vi "9203_UI.vi"(8 "error in (no error)":errorcluster, 11 "Node Ptr":T2 format="%.0x") -> (0 "error out":errorcluster)   [LabVIEW 2017, in "Modules.lvlib" / "9203.lvclass"]
uses:
  9203.lvclass
  <vilib>/NI Veristand/Custom Device API/Custom Device Item Ref.ctl
  RSI Module/SubPanel Command.ctl
  C:/Users/dbuck/Documents/GitHub/Scan-Engine-Custom-Device-Classes/Source/RSI Module/RSI Module.lvclass
  9203.lvclass/9203.ctl
  Range.ctl
  RSI Module/RSI Module.lvclass
  <vilib>/NI Veristand/Custom Device API/Custom Device API.lvlib
panel:
  out "_SupportedRanges":string[][](array[string])=[["+/- 20mA", "0-20 mA"], ["+/- 20mA", "0-20 mA"], ["+/- 20mA", "0-20 mA"], ["+/- 20mA", "0-20 mA"], ["+/- 20mA", "0-20 mA"], ["+/- 20mA", "0-20 mA"], ["+/- 20mA", "0-20 mA"], ["+/- 20mA", "0-20 mA"]]
  in  "_Update Chan Settings":bool
  in  "_Update Ring Controls":bool
  in  "_Input Ranges":T1(array[ring])=[enum."+/- 10V", enum."+/- 10V", enum."+/- 10V", enum."+/- 10V", enum."+/- 10V", enum."+/- 10V", enum."+/- 10V", enum."+/- 10V", enum."+/- 10V", enum."+/- 10V", enum."+/- 10V", enum."+/- 10V", enum."+/- 10V", enum."+/- 10V", enum."+/- 10V", enum."+/- 10V", enum."+/- 10V", enum."+/- 10V", enum."+/- 10V", enum."+/- 10V", enum."+/- 10V", enum."+/- 10V", enum."+/- 10V", enum."+/- 10V", enum."+/- 10V", enum."+/- 10V", enum."+/- 10V", enum."+/- 10V", enum."+/- 10V", enum."+/- 10V", enum."+/- 10V", enum."+/- 10V"]
  in  "Input Range":u16(ring) items=["+/- 20mA", "0-20 mA"]
  in  "Channels":i32[](listbox)=[0]
  in  "SubPanel Event":refnum<user-event>
  in  "Header":cluster{"Section Name":string}={"Section Name"="NI 9205 Settings"}
  # "Channel Configuration"
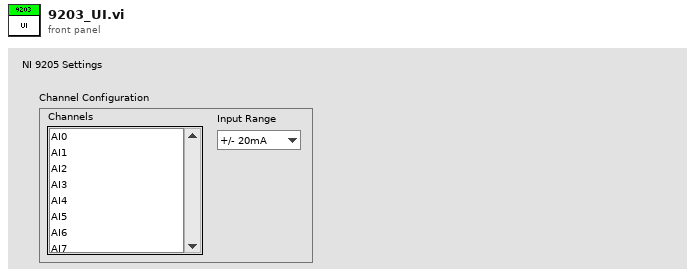
[diagram p1: front panel]
types:
  T1 = enum8{"+/- 10V", "+/- 5V", "+/- 1V", "+/- 200mV"}[]
  T2 = typedef "Custom Device API.lvlib/Custom Device Item Ref.ctl" = u64
  T3 = typedef "Modules.lvlib/9203.lvclass/Channel Settings.ctl" = cluster{"Range":T4}[]
  T4 = typedef "Modules.lvlib/9203.lvclass/Range.ctl" = u32
  T5 = typedef "Modules.lvlib/RSI Module.lvclass/Module Models.ctl" = enum16{"Empty", "NI 9201", "NI 9203", "NI 9205", "NI 9206", "NI 9207", "NI 9208", "NI 9211", "NI 9212", "NI 9213", "NI 9214", "NI 9215", "NI 9217", "NI 9219", "NI 9220", "NI 9221", "NI 9222", "NI 9223", "NI 9225", "NI 9227", "NI 9229", "NI 9233", "NI 9234", "NI 9235", "NI 9236", "NI 9237", "NI 9239", "NI 9242", "NI 9244", "NI 9263", "NI 9264", "NI 9265", "NI 9269", "NI 9375", "NI 9401", "NI 9402", "NI 9403", "NI 9411", "NI 9421", "NI 9422", "NI 9423", "NI 9425", "NI 9426", "NI 9435", "NI 9437", "NI 9472", "NI 9474", "NI 9475", "NI 9476", "NI 9477", "NI 9478", "NI 9481", "NI 9482", "NI 9485"}
  T6 = typedef "Modules.lvlib/RSI Module.lvclass/SubPanel Command.ctl" = enum16{"Stop"}
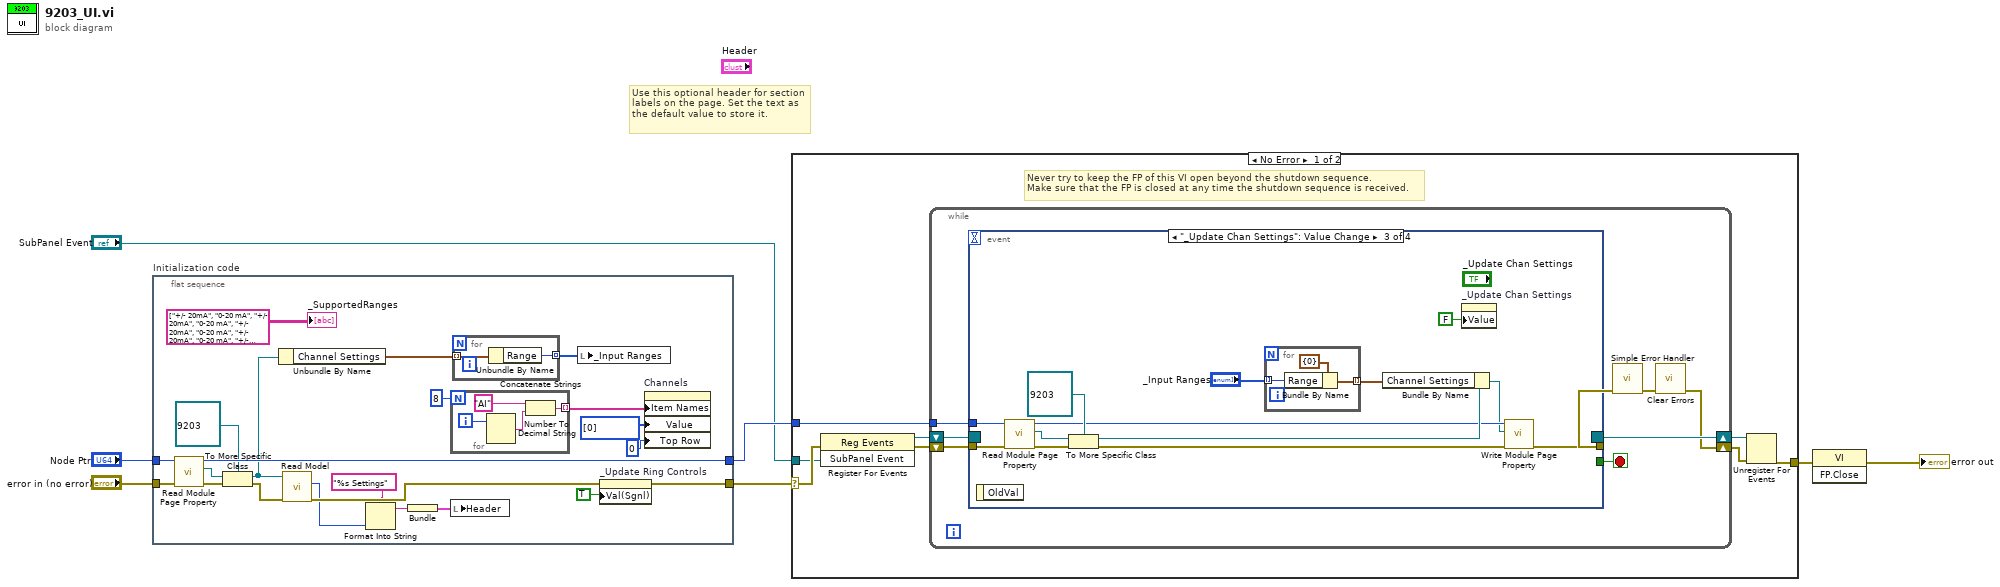
[diagram p0: block diagram]
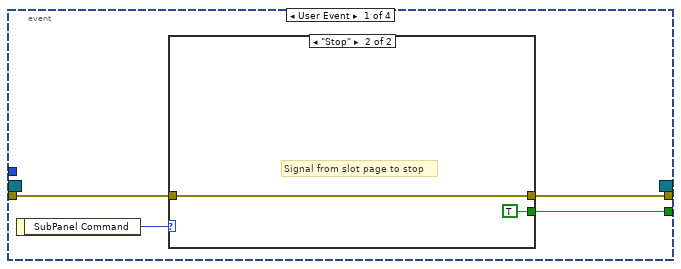
[diagram p2: hidden frame]
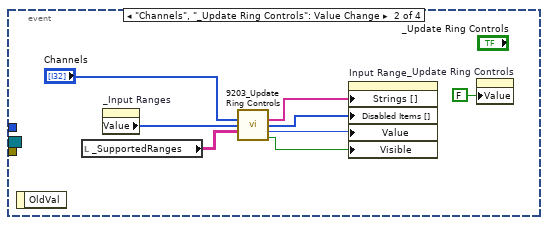
[diagram p4: hidden frame]
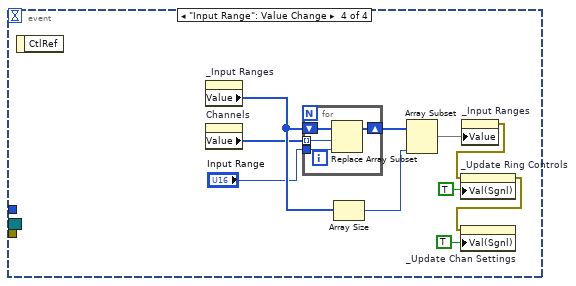
[diagram p5: hidden frame]
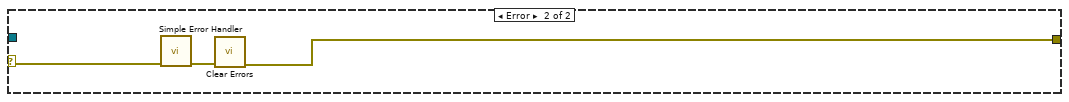
[diagram p6: hidden frame]
diagram:
  # "Use this optional header for section labels on the page. Set the text as the default value to store it."
  n1 = flat-sequence "Initialization code" {
    tunnel: "error in (no error)" -> [w28]
    tunnel: "Node Ptr" -> [w29]
    tunnel: [w17] -> w1
    tunnel: [w27] -> w4
    frame #0 {
      n2 = call "Read Module Page Property.vi"("error in (no error)"=w28, "Node Ptr In"=w29) -> ("error out"=w26:errorcluster, "RSI Module"=w24:refnum<class "RSI Module.lvclass">, "Node Ptr Out"=w27:T2)  [unwired: 7 in]
      n3 = To More Specific Class(target class=refnum<class "9203.lvclass"> refnum ("9205 in"), reference=w24, error in=w26) -> (specific class reference=w16:refnum<class "9203.lvclass">, error out=w15:errorcluster)
      n4 = Unbundle By Name(w16) -> ("Channel Settings"=w18:T3)
      n5 = call "Read Model.vi"("error in (no error)"=w15, "RSI Module in"=w16) -> ("error out"=w14:errorcluster, "Model"=w12:T5)  [unwired: 7 in, 1 out]
      n6 = Format Into String(format string="%s Settings", w12) -> (resulting string=w10:string)  [unwired: 2 in, 1 out]
      n7 = Bundle(w10) -> (w13:cluster{string})  [unwired: 1 in]
      n8 = for {
        N: 8 -> [_]
        tunnel: [w32] -> w23 mode=indexing
        i -> [w34]
        n9 = Number To Decimal String(number=w34) -> (decimal integer string=w33:string)  [unwired: 1 out]
        n10 = Concatenate Strings("AI", w33) -> (w32:string)
      }
      n11 = local write "Header"(w13) -> ()
      n12 = for {
        tunnel: w18 -> [w31] mode=indexing
        tunnel: [w30] -> w21 mode=indexing
        n13 = Unbundle By Name(w31) -> ("Range"=w30:T4)
      }
      n14 = local write "_Input Ranges"(w21) -> ()
      n15 = property on="_Update Ring Controls" class="Bool (strict)"(error in=w14, "Val(Sgnl)"=TRUE ("Value (Signaling)")) -> (error out=w17:errorcluster)  [unwired: 1 in, 1 out]
      n16 = property on="Channels" class="LstBox (strict)"("Item Names"=w23, "Value"=i32[] [0] ("Channels"), "Top Row"=0) -> ()  [unwired: 2 in, 2 out]
      "_SupportedRanges" <- string[][] [["+/- 20mA", "0-20 mA"], ["+/- 20mA", "0-20 mA"], ["+/- 20mA", "0-20 mA"], ["+/- 20mA", "0-20 mA"], ["+/- 20mA", "0-20 mA"], ["+/- 20mA", "0-20 mA"], ["+/- 20mA", "0-20 mA"], ["+/- 20mA", "0-20 mA"]] ("Ranges")
    }
  }
  n17 = case shown="No Error" w1 {
    selector: w1 -> [w37 w99]
    tunnel: [w41 w97] -> w7
    tunnel: w4 -> [w38 _]
    tunnel: "SubPanel Event" -> [w36 _]
    frame No Error {
      # "Never try to keep the FP of this VI open beyond the shutdown sequence.\nMake sure that the FP is closed at any time the shutdown sequence is received."
      n18 = register-events(error in=w37, w36) -> (reference out=w39:refnum<event-registration>, error out=w40:errorcluster)  [unwired: 1 in]
      n19 = while {
        tunnel: w38 -> [w47]
        shift-right: [w44] -> w42
        shift-left: w40 -> [w50]
        shift-right: [w51] -> w43
        shift-left: w39 -> [w49]
        stop <- w48 stop-if-true
        n20 = event shown="[2] \"_Update Chan Settings\": Value Change" {
          selector: w49 -> [_ _ _ _]
          dyn-events: [_ _ _ _] -> w51
          timeout: _ -> [_ _ _ _]
          tunnel: w50 -> [w54 _ w71 _]
          tunnel: [w53 _ _ _] -> w48
          tunnel: [w52 _ w70 _] -> w46
          tunnel: w47 -> [_ _ w72 _]
          event User Event {
            n21 = event-data() -> ("SubPanel Command"=w55:T6)  [unwired: 1 out]
            n22 = case shown="\"Stop\"" w55 {
              tunnel: w54 -> [w56 w57]
              tunnel: [w56 w57] -> w52
              tunnel: [_ TRUE] -> w53
              frame Default {
              }
              frame "Stop" {
                # "Signal from slot page to stop"
              }
            }
          }
          event "Channels", "_Update Ring Controls": Value Change {
            n23 = event-data() -> ()  [unwired: 2 out]
            n24 = local read "_SupportedRanges"() -> (w64:string[][])
            n25 = property on="_Input Ranges" class="Arr (strict)"() -> ("Value"=w65:T1)  [unwired: 2 in, 2 out]
            n26 = call "9203_Update Ring Controls.vi"("SelectedChannels"="Channels", "ChannelConfig"=w65, "SupportedModes"=w64) -> ("Strings out"=w63:string[], "Disabled Items out"=w62:i32[], "Value out"=w61:u8, "Visible out"=w60:bool)  [unwired: 9 in]
            n27 = property on="Input Range" class="Ring (strict)"("Strings []"=w63, "Disabled Items []"=w62, "Value"=w61, "Visible"=w60) -> ()  [unwired: 2 in, 2 out]
            n28 = property on="_Update Ring Controls" class="Bool (strict)"("Value"=FALSE ("_Update Ring Controls 2")) -> ()  [unwired: 2 in, 2 out]
          }
          event "_Update Chan Settings": Value Change {
            n29 = event-data() -> ()  [unwired: 2 out]
            n30 = call "Read Module Page Property.vi"("error in (no error)"=w71, "Node Ptr In"=w72) -> ("error out"=w77:errorcluster, "RSI Module"=w78:refnum<class "RSI Module.lvclass">, "Node Ptr Out"=w74:T2)  [unwired: 7 in]
            n31 = To More Specific Class(target class=refnum<class "9203.lvclass"> refnum ("9205 in"), reference=w78, error in=w77) -> (specific class reference=w76:refnum<class "9203.lvclass">, error out=w75:errorcluster)
            n32 = for {
              tunnel: "_Input Ranges" -> [w82] mode=indexing
              tunnel: [w81] -> w67 mode=indexing
              n33 = Bundle By Name(cluster=cluster{"Range":T4} {"Range"=0}, "Range"=w82) -> (w81:cluster{"Range":T4})
            }
            n34 = Bundle By Name(cluster=w76, "Channel Settings"=w67) -> (w73:refnum<class "9203.lvclass">)
            n35 = property on="_Update Chan Settings" class="Bool (strict)"("Value"=FALSE ("_Update Values")) -> ()  [unwired: 2 in, 2 out]
            n36 = call "Write Module Page Property.vi"("error in (no error)"=w75, "RSI Module"=w73, "Node Ptr In"=w74) -> ("error out"=w70:errorcluster)  [unwired: 6 in, 2 out]
          }
          event "Input Range": Value Change {
            n37 = event-data() -> ()  [unwired: 2 out]
            n38 = property on="_Input Ranges" class="Arr (strict)"() -> ("Value"=w86:T1)  [unwired: 2 in, 2 out]
            n39 = property on="Channels" class="LstBox (strict)"() -> ("Value"=w83:i32[])  [unwired: 2 in, 2 out]
            n40 = for {
              tunnel: "Input Range" -> [w95]
              tunnel: w83 -> [w93] mode=indexing
              shift-right: [w94] -> w85
              shift-left: w86 -> [w96]
              n41 = Replace Array Subset(array=w96, new element=w95, index=w93) -> (w94:T1)
            }
            n42 = Array Size(array=w86) -> (size(s)=w92:i32)
            n43 = Array Subset(array=w85, length=w92) -> (w91:T1)  [unwired: 1 in]
            n44 = property on="_Input Ranges" class="Arr (strict)"("Value"=w91) -> (error out=w89:errorcluster)  [unwired: 2 in, 1 out]
            n45 = property on="_Update Ring Controls" class="Bool (strict)"(error in=w89, "Val(Sgnl)"=TRUE ("Value (Signaling)")) -> (error out=w87:errorcluster)  [unwired: 1 in, 1 out]
            n46 = property on="_Update Chan Settings" class="Bool (strict)"(error in=w87, "Val(Sgnl)"=TRUE ("Value (Signaling)")) -> ()  [unwired: 1 in, 2 out]
          }
        }
        n47 = call <vilib>:"Simple Error Handler.vi"("error in (no error)"=w46) -> ("error out"=w45:errorcluster)  [unwired: 1 in, 7 out]
        n48 = call <vilib>:"Clear Errors.vi"("error in (no error)"=w45) -> ("error out"=w44:errorcluster)  [unwired: 1 in, 5 out]
      }
      n49 = Unregister For Events(event registration refnum=w43, error in=w42) -> (error out=w41:errorcluster)
    }
    frame Error {
      n50 = call <vilib>:"Simple Error Handler.vi"("error in (no error)"=w99) -> ("error out"=w98:errorcluster)  [unwired: 1 in, 7 out]
      n51 = call <vilib>:"Clear Errors.vi"("error in (no error)"=w98) -> ("error out"=w97:errorcluster)  [unwired: 1 in, 5 out]
    }
  }
  n52 = invoke class="VI" method="FP.Close"(error in=w7) -> (error out=→"error out":errorcluster)  [unwired: 2 in, 2 out]
